vi "3D加速度传感器实验.vi"() -> ()   [LabVIEW 2011]
uses:
  <vilib>/STM32_DriverVI_Interface_F4/IIC/IIC_Select_F4.ctl
  <vilib>/STM32_DriverVI_Interface_F4/LCD/Show_Mode_F4.ctl
  <vilib>/STM32_DriverVI_Interface_F4/LCD/Font_Size_F4.ctl
  <vilib>/STM32_DriverVI_Interface_F4/LCD/Brush Color_Index_F4.ctl
  <vilib>/eio/EIO_TerminalDirection.ctl
  <vilib>/STM32_DriverVI_Interface_F4/LCD/LCD_Init_F4.vi
  <vilib>/STM32_DriverVI_Interface_F4/GPIO_EIO/GPO_EIO_Inner_F4.vi
  <vilib>/eio/EIONode/EIONode.xnode
panel:
  out "Z_Angle(°)":dbl
  out "Y_Angle(°)":dbl
  out "X_Angle(°)":dbl
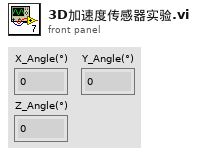
[diagram p1: front panel]
types:
  T1 = enum8{"P0", "P1", "P2", "P3", "P4", "P5", "P6", "P7", "P8", "P9", "P10", "P11", "P12", "P13", "P14", "P15"}
  T2 = enum8{"Port_A", "Port_B", "Port_C", "Port_D", "Port_E", "Port_F", "Port_G", "Port_H", "Port_I"}
  T3 = typedef "IIC_Select_F4.ctl" = enum8{"IIC_Group_1", "IIC_Group_2", "IIC_Group_3", "IIC_Group_4", "IIC_Group_5", "IIC_Group_6", "IIC_Group_7", "IIC_Group_8"}
  T4 = typedef "Show_Mode_F4.ctl" = enum8{"非叠加显示", "叠加显示"}
  T5 = typedef "Font_Size_F4.ctl" = enum8{"Small_Font（12）", "Big_Font（16）"}
  T6 = typedef "Brush Color_Index_F4.ctl" = enum8{"White", "Black", "Blue", "Green_Blue", "Red", "Magenta（品红）", "Green", "Cyan（青色）", "Yellow", "Brown", "Brown_Red", "Gray", "Dark_Blue", "Light_Blue", "Gray_Blue", "Light_Green", "Light_Gray", "Light_Gray_Blue", "Light_Brown_Blue"}
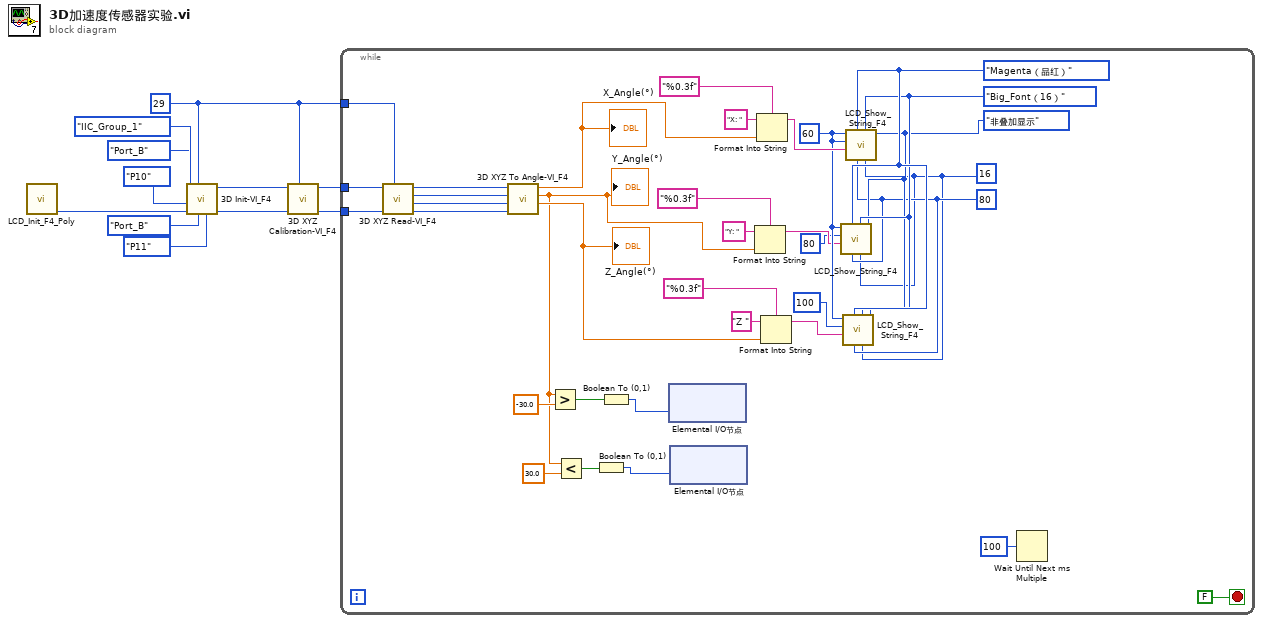
[diagram p0: block diagram]
diagram:
  w1 = u8 29 ("器件地址（7位）")
  n1 = call-poly <vilib>:"LCD_Init_F4_Poly.vi"() -> ("err_out"=w11:u8)  [unwired: 10 in, 1 out]
  n2 = call <vilib>:"3D Init-VI_F4.vi"("SDA_pin"=T1."P11", "SDA_PortX"=T2."Port_B", "器件地址（7位）"=w1, "err_in"=w11, "SCL_pin"=T1."P10", "SCL_PortX"=T2."Port_B", "IIC_Select"=IIC_Select_F4."IIC_Group_1") -> ("err_out"=w5:u8, "IIC_Reference_Out"=w4:u16)  [unwired: 1 in, 2 out]
  n3 = call <vilib>:"3D XYZ Calibration-VI_F4.vi"("器件地址（7位）"=w1, "err_in"=w5, "IIC_Reference_In"=w4) -> ("err_out"=w3:u8, "IIC_Reference_Out"=w2:u16)  [unwired: 7 in]
  n4 = while {
    tunnel: w3 -> [w46]
    tunnel: w2 -> [w45]
    tunnel: w1 -> [w44]
    stop <- FALSE stop-if-true
    w31 = u16 60 ("X_Position")
    w22 = u16 80 ("Width")
    w21 = u16 16 ("Height")
    w23 = Show_Mode_F4."非叠加显示" ("Show_Mode")
    w24 = Font_Size_F4."Big_Font（16）" ("Font_Size")
    w25 = Brush_Color_Index_F4."Magenta（品红）" ("Brush Color")
    n5 = call <vilib>:"3D XYZ Read-VI_F4.vi"("器件地址（7位）"=w44, "err_in"=w46, "IIC_Reference_In"=w45) -> ("err_out"=w43:u8, "Z（-4096~4095）"=w40:i16, "Y（-4096~4095）"=w41:i16, "X（-4096~4095）"=w42:i16)  [unwired: 4 in, 1 out]
    n6 = call <vilib>:"3D XYZ To Angle-VI_F4.vi"("err_in"=w43, "Z（-4096~4095）"=w40, "Y（-4096~4095）"=w41, "X（-4096~4095）"=w42) -> ("Z_Angle(°)"=w26:dbl, "Y_Angle(°)"=w16:dbl, "X_Angle(°)"=w39:dbl)  [unwired: 4 in, 1 out]
    "X_Angle(°)" <- w39
    "Y_Angle(°)" <- w16
    "Z_Angle(°)" <- w26
    n7 = Greater?(x=w16, y=-30.0) -> (0:w15:bool)
    n8 = Less?(x=w16, y=30.0) -> (x < y?=w13:bool)
    n9 = Boolean To (0,1)(Boolean=w13) -> (0, 1=w12:i16)
    n10 = Boolean To (0,1)(Boolean=w15) -> (0, 1=w14:i16)
    n11 = xnode "Elemental I/O节点"("LED_1"=w14) -> ()  [unwired: 1 in, 1 out]
    n12 = xnode "Elemental I/O节点"("LED_2"=w12) -> ()  [unwired: 1 in, 1 out]
    n13 = Format Into String(format string="%0.3f" ("格式字符串"), initial string="Y: " ("初始字符串"), w16) -> (resulting string=w30:string)  [unwired: 1 in, 1 out]
    n14 = Format Into String(format string="%0.3f" ("格式字符串"), initial string="X: " ("初始字符串"), w39) -> (resulting string=w36:string)  [unwired: 1 in, 1 out]
    n15 = Format Into String(format string="%0.3f" ("格式字符串"), initial string="Z " ("初始字符串"), w26) -> (resulting string=w27:string)  [unwired: 1 in, 1 out]
    n16 = call <vilib>:"LCD_Show_String_F4.vi"("Show_Mode"=w23, "Height"=w21, "Font_Size"=w24, "Width"=w22, "Brush Color"=w25, "String"=w30, "Y_Position"=u16 80, "X_Position"=w31) -> ()  [unwired: 3 in, 1 out]
    n17 = call <vilib>:"LCD_Show_String_F4.vi"("Show_Mode"=w23, "Height"=w21, "Font_Size"=w24, "Width"=w22, "Brush Color"=w25, "String"=w27, "Y_Position"=u16 100, "X_Position"=w31) -> ()  [unwired: 3 in, 1 out]
    n18 = call <vilib>:"LCD_Show_String_F4.vi"("Show_Mode"=w23, "Height"=w21, "Font_Size"=w24, "Width"=w22, "Brush Color"=w25, "String"=w36, "Y_Position"=w31, "X_Position"=w31) -> ()  [unwired: 3 in, 1 out]
    n19 = Wait Until Next ms Multiple(millisecond multiple=u32 100 ("毫秒倍数")) -> ()  [unwired: 1 out]
  }
